vi "Start Channel.vi"(0 "Potentiostat Galvanostat in":refnum<class "Potentiostat Galvanostat.lvclass">, 11 "error in (no error)":errorcluster) -> (4 "Potentiostat Galvanostat out":refnum<class "Potentiostat Galvanostat.lvclass">, 15 "error out":errorcluster)   [LabVIEW 2018, in "Potentiostat Galvanostat.lvclass"]
uses:
  Potentiostat Galvanostat.lvclass
  Potentiostat Galvanostat.lvclass/Potentiostat Galvanostat.ctl
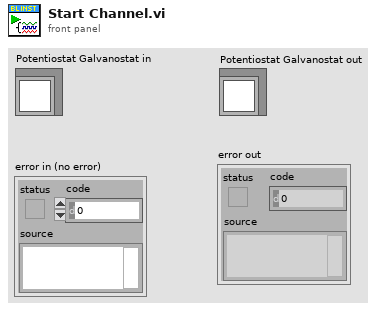
[diagram p1: front panel]
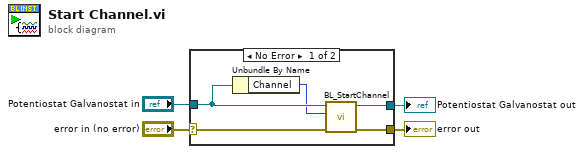
[diagram p0: block diagram]
diagram:
  n1 = case shown="No Error" "error in (no error)" {
    selector: "error in (no error)" -> [w9 w11]
    tunnel: [w8 w11] -> w3
    tunnel: [w5 w10] -> w1
    tunnel: "Potentiostat Galvanostat in" -> [w7 w10]
    frame No Error {
      n2 = Unbundle By Name(w7) -> ("Channel"=w6:u8)
      n3 = call-dynamic "BL_StartChannel.vi"("error in (no error)"=w9, "Channel"=w6, "Potentiostat Galvanostat in"=w7) -> ("error out"=w8:errorcluster, "Potentiostat Galvanostat out"=w5:refnum<class "Potentiostat Galvanostat.lvclass">)  [unwired: 6 in, 1 out]
    }
    frame Error {
    }
  }
  "error out" <- w3
  "Potentiostat Galvanostat out" <- w1
